vi "hmp4000 Configure Channel.vi"(8 "error in (no error)":errorcluster, 9 "Channel (Channel 1)":i32(ring)=1 items=["Channel 1"=1, "Channel 2"=2, "Channel 3"=3, "Channel 4"=4], 11 "VISA resource name":refnum<visa-resource-name>) -> (0 "error out":errorcluster, 3 "VISA resource name out":refnum<visa-resource-name>)   [LabVIEW 2022 SP3]
doc: "This VI selects the channels. All the following channel-selective commands will be applied for this channel.\n\nAttribute:\nHMP4000_ATTR_SELECTION_OF_CHANNEL\n\nRemote-control command:\nINSTrument:SELect OUTPut1 | OUTPut2 | OUTPut3 | OUTPut4"
uses:
  Instance           1 33Saved   hmp4000 Configure Channel .vi
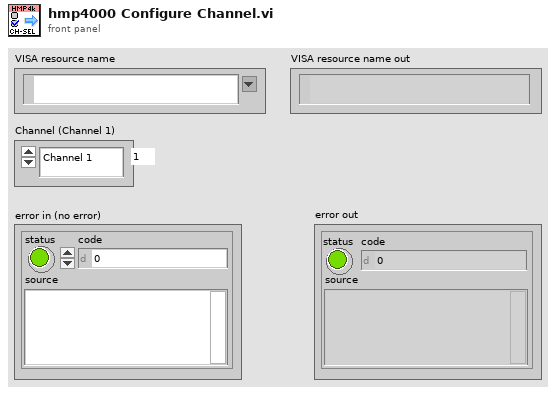
[diagram p1: front panel]
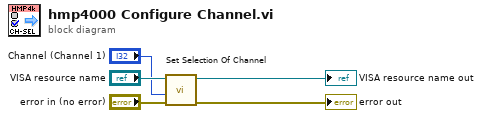
[diagram p0: block diagram]
diagram:
  n1 = call "Set Selection Of Channel"("error in (no error)"="error in (no error)", "Selection Of Channel (0 - <UNDEFINED>)"="Channel (Channel 1)", "instrument handle"="VISA resource name") -> ("error out"=→"error out":errorcluster, "instrument handle out"=→"VISA resource name out":refnum<visa-resource-name>)  [unwired: 7 in]
